vi "contains.vi"(0 "reference":refnum<class "GeneralPathEdge.lvclass">, 1 "point2D":T1 {"y" format="%.2f"; "x" format="%.2f"}, 2 "GraphicsRef":refnum<class "Graphics.lvclass">, 5 "error in (no error)":errorcluster) -> (14 "reference out":refnum<class "GeneralPathEdge.lvclass">, 15 "contains":bool, 19 "error out":errorcluster)   [LabVIEW 2016, in "GeneralPathEdge.lvclass"]
doc: "public boolean contains(Point2D aPoint)\n {\n final double MAX_DIST = 3;\n\n // the end points may contain small nodes, so don't\n // match them\n Line2D conn = getConnectionPoints();\n if (aPoint.distance(conn.getP1()) <= MAX_DIST \n || aPoint.distance(conn.getP2()) <= MAX_DIST)\n return false;\n\n GeneralPath p = getPath();\n BasicStroke fatStroke = new BasicStroke(\n (float)(2 * MAX_DIST));\n Shape fatPath = fatStroke.createStrokedShape(p);\n return fatPath.contains(aPoint);\n }"
uses:
  <resource>/Framework/Providers/Open_GDS/UML/GeneralPathEdge_class/GeneralPathEdge.lvclass
  C:/Program Files (x86)/National Instruments/LabVIEW 2016/resource/Framework/Providers/Open_GDS/UML/AbstractEdge_class/AbstractEdge.lvclass
  <resource>/Framework/Providers/Open_GDS/UML/General/Point/Point Point2D.ctl
  <resource>/Framework/Providers/Open_GDS/UML/Graphics_class/Graphics.lvclass
  <resource>/Framework/Providers/Open_GDS/UML/AbstractEdge_class/AbstractEdge.lvclass
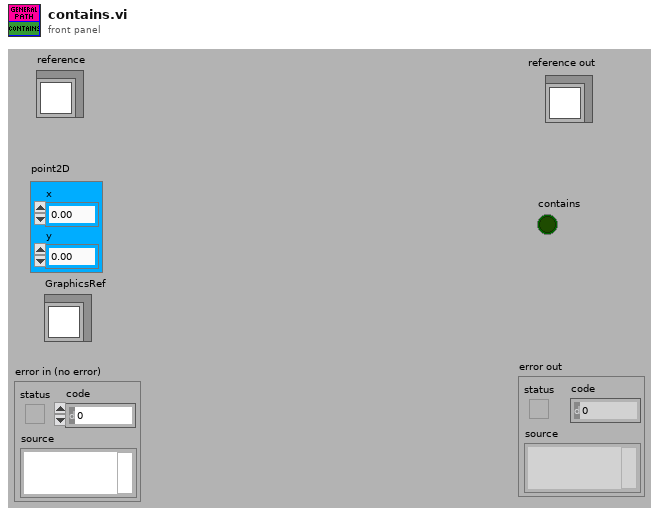
[diagram p1: front panel]
types:
  T1 = typedef "Point Point2D.ctl" = cluster{"x":dbl, "y":dbl}
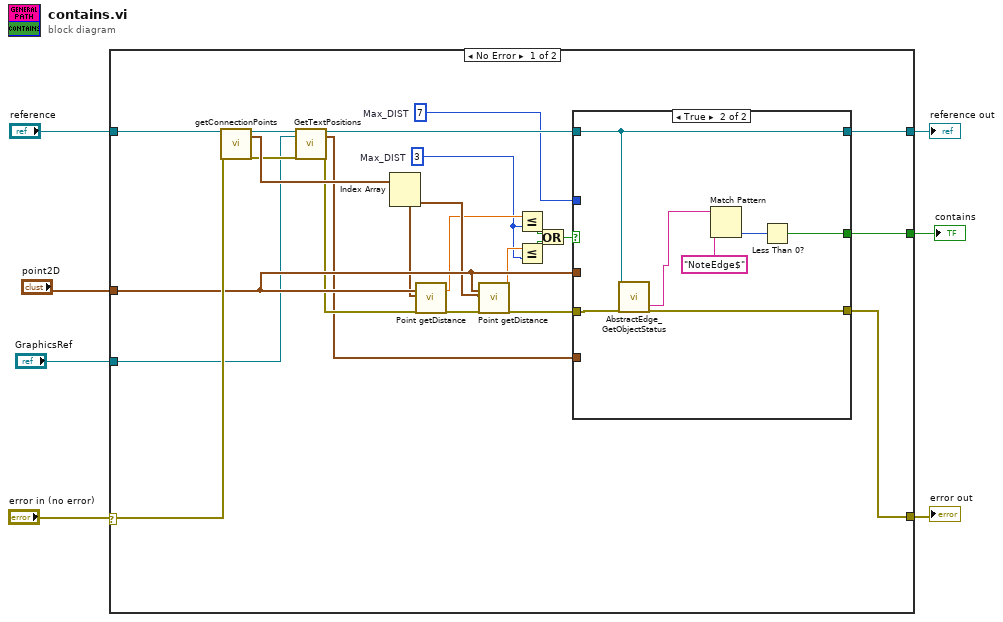
[diagram p0: block diagram]
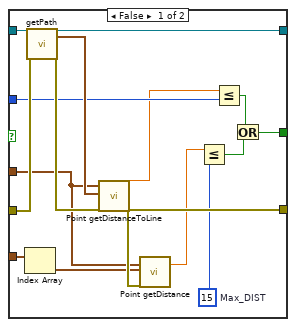
[diagram p2: hidden frame]
diagram:
  n1 = case shown="No Error" "error in (no error)" {
    selector: "error in (no error)" -> [w28 w55]
    tunnel: "reference" -> [w31 w56]
    tunnel: [w30 w55] -> w6
    tunnel: [w29 w56] -> w5
    tunnel: [w27 _] -> w3
    tunnel: "point2D" -> [w26 _]
    tunnel: "GraphicsRef" -> [w8 _]
    frame No Error {
      w10 = 7  # Max_DIST
      w11 = 3  # Max_DIST
      n2 = call-dynamic "getConnectionPoints.vi"("reference"=w31, "error in (no error)"=w28) -> ("reference out"=w15:refnum<class "GeneralPathEdge.lvclass">, "connectionPoints"=w25:T1[], "error out"=w13:errorcluster)  [unwired: 15 in]
      n3 = call-dynamic "GetTextPositions.vi"("reference"=w15, "GraphicsRef"=w8, "error in (no error)"=w13) -> ("reference out"=w14:refnum<class "GeneralPathEdge.lvclass">, "connectionPoints"=w9:T1[], "error out"=w12:errorcluster)  [unwired: 14 in]
      n4 = Index Array(array=w25) -> (element #1=w23:T1, element #2=w22:T1)  [unwired: 2 in]
      n5 = call <resource>:"Point getDistance.vi"("point1"=w26, "point2"=w23, "error in (no error)"=w12) -> ("distance"=w20:dbl, "error out"=w24:errorcluster)  [unwired: 15 out]
      n6 = call <resource>:"Point getDistance.vi"("point1"=w26, "point2"=w22, "error in (no error)"=w24) -> ("distance"=w21:dbl, "error out"=w16:errorcluster)  [unwired: 15 out]
      n7 = Less Or Equal?(x=w20, y=w11) -> (x <= y?=w19:bool)
      n8 = Less Or Equal?(x=w21, y=w11) -> (x <= y?=w18:bool)
      n9 = Or(x=w19, y=w18) -> (x .or. y?=w17:bool)
      n10 = case shown="True" w17 {
        tunnel: [w33 w49] -> w27
        tunnel: w14 -> [w47 w53]
        tunnel: w16 -> [w46 w54]
        tunnel: w26 -> [w39 _]
        tunnel: w10 -> [w43 _]
        tunnel: [w41 w53] -> w29
        tunnel: [w40 w52] -> w30
        tunnel: w9 -> [w38 _]
        frame False {
          w34 = 15  # Max_DIST
          n11 = Index Array(array=w38) -> (element=w37:T1)  [unwired: 1 in]
          n12 = call-dynamic "getPath.vi"("reference"=w47, "error in (no error)"=w46) -> ("reference out"=w41:refnum<class "GeneralPathEdge.lvclass">, "points"=w44:T1[], "error out"=w45:errorcluster)  [unwired: 15 in]
          n13 = call <resource>:"Point getDistanceToLine.vi"("point1"=w39, "line"=w44, "error in (no error)"=w45) -> ("minDistance"=w36:dbl, "error out"=w40:errorcluster)  [unwired: 15 out]
          n14 = call <resource>:"Point getDistance.vi"("point1"=w39, "point2"=w37, "error in (no error)"=w40) -> ("distance"=w35:dbl)  [unwired: 16 out]
          n15 = Less Or Equal?(x=w35, y=w34) -> (x <= y?=w32:bool)
          n16 = Less Or Equal?(x=w36, y=w43) -> (x <= y?=w42:bool)
          n17 = Or(x=w42, y=w32) -> (x .or. y?=w33:bool)
        }
        frame True {
          n18 = call <resource>:"AbstractEdge_GetObjectStatus.vi"("reference in"=w53, "error in (no error)"=w54) -> ("Class name"=w48:string, "error out"=w52:errorcluster)  [unwired: 16 out]
          n19 = Match Pattern(string=w48, regular expression="NoteEdge$") -> (offset past match=w50:i32)  [unwired: 4 out]
          n20 = Less Than 0?(x=w50) -> (x < 0?=w49:bool)
        }
      }
    }
    frame Error {
    }
  }
  "reference out" <- w5
  "error out" <- w6
  "contains" <- w3
